vi "LoadConfigFile.vi"(0 "error in (no error)":errorcluster) -> (20 "error out":errorcluster, 21 "IP":string caption="Robot IP Address", 22 "Licensee":string, 23 "Key":string, 24 "Username":string, 25 "Password":string)   [LabVIEW 2023]
uses:
  <vilib>/Utility/config.llb/NI_LVConfig.lvlib
  <vilib>/Utility/config.llb/Read Key (String).vi
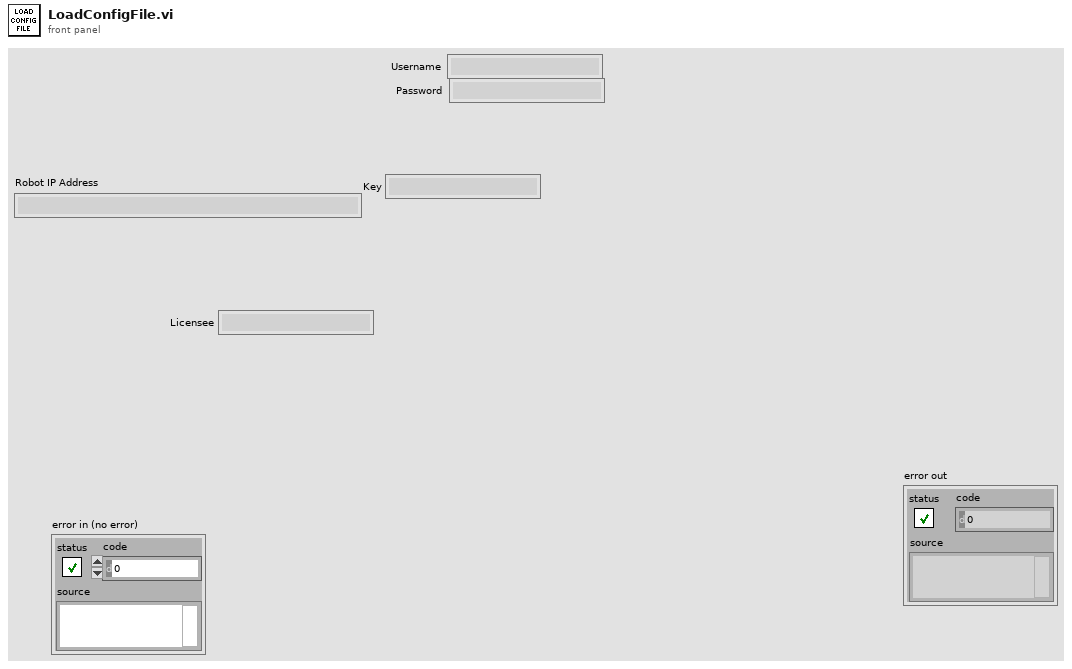
[diagram p1: front panel]
types:
  T1 = typedef "NI_LVConfig.lvlib/Config Data RefNum.ctl" = refnum<k1>
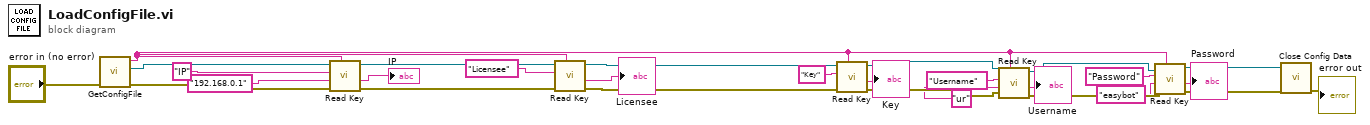
[diagram p0: block diagram]
diagram:
  n1 = call "GetConfigFile.vi"("error in (no error)"="error in (no error)") -> ("error out"=w27:errorcluster, "refnum"=w26:T1, "section"=w1:string)  [unwired: 8 in]
  n2 = call-poly <vilib>:"Read Key.vi"("section"=w1, "error in (no error)"=w27, "default value"="192.168.0.1", "key"="IP", "refnum"=w26) -> ("error out"=w15:errorcluster, "value"=→"IP":string, "refnum out"=w14:T1)  [unwired: 3 in, 1 out]
  n3 = call-poly <vilib>:"Read Key.vi"("section"=w1, "error in (no error)"=w15, "key"="Licensee", "refnum"=w14) -> ("error out"=w22:errorcluster, "value"=→"Licensee":string, "refnum out"=w23:T1)  [unwired: 4 in, 1 out]
  n4 = call-poly <vilib>:"Read Key.vi"("section"=w1, "error in (no error)"=w22, "key"="Key", "refnum"=w23) -> ("error out"=w9:errorcluster, "value"=→"Key":string, "refnum out"=w6:T1)  [unwired: 4 in, 1 out]
  n5 = call-poly <vilib>:"Read Key.vi"("section"=w1, "error in (no error)"=w9, "default value"="ur", "key"="Username", "refnum"=w6) -> ("error out"=w8:errorcluster, "value"=→"Username":string, "refnum out"=w5:T1)  [unwired: 3 in, 1 out]
  n6 = call-poly <vilib>:"Read Key.vi"("section"=w1, "error in (no error)"=w8, "default value"="easybot", "key"="Password", "refnum"=w5) -> ("error out"=w7:errorcluster, "value"=→"Password":string, "refnum out"=w4:T1)  [unwired: 3 in, 1 out]
  n7 = call <vilib>:"Close Config Data.vi"("error in (no error)"=w7, "refnum"=w4) -> ("error out"=→"error out":errorcluster)  [unwired: 8 in, 1 out]
